vi "New Motion Profile.vi"(7 "Time Between Points (ms)":dbl=20.0, 8 "error in (no error)":errorcluster, 10 "Starting Conditions":T1, 11 "Control Boundaries":T2) -> (0 "error out":errorcluster, 3 "Motion Profile Generator out":refnum<class "Motion Profile Generator.lvclass">)   [LabVIEW 2019, in "Motion Profile Generator.lvclass"]
uses:
  Motion Profile Generator.lvclass
  Type Defs/Control Boundaries.ctl
  Type Defs/Motion Snapshot.ctl
  Motion Profile Generator.lvclass/Motion Profile Generator.ctl
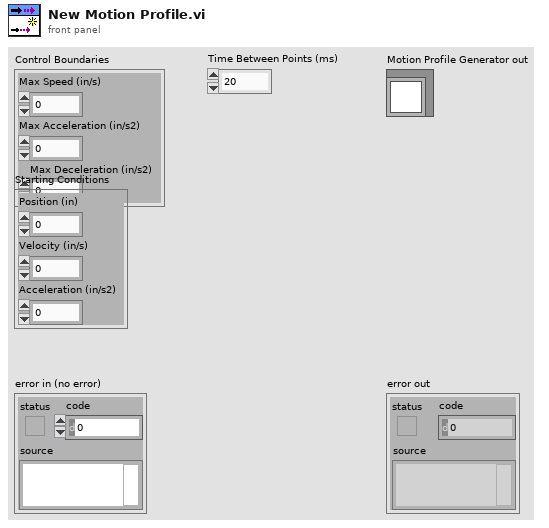
[diagram p1: front panel]
types:
  T1 = typedef "Motion Profile Generator.lvclass/Motion Snapshot.ctl" = cluster{"Position (in)":dbl, "Velocity (in/s)":dbl, "Acceleration (in/s2)":dbl}
  T2 = typedef "Motion Profile Generator.lvclass/Control Boundaries.ctl" = cluster{"Max Speed (in/s)":dbl, "Max Acceleration (in/s2)":dbl, "Max Deceleration (in/s2)":dbl}
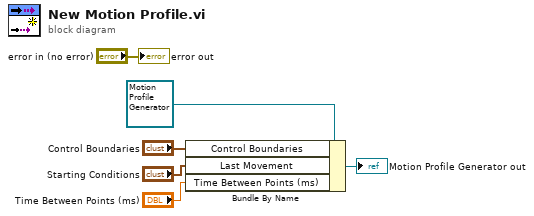
[diagram p0: block diagram]
diagram:
  n1 = Bundle By Name(cluster=refnum<class "Motion Profile Generator.lvclass"> refnum ("Motion Profile Generator in"), "Control Boundaries"="Control Boundaries", "Last Movement"="Starting Conditions", "Time Between Points (ms)"="Time Between Points (ms)") -> (→"Motion Profile Generator out":refnum<class "Motion Profile Generator.lvclass">)
  "error out" <- "error in (no error)"
